vi "Stamp interface.vi"(4 "intercept":dbl=46.7 format="%.2f", 6 "slope":dbl=1.91 format="%.2f", 10 "Controls":T1 {"Pump speed" format="%.2f"}, 11 "Serial Port":refnum<visa-resource-name>) -> (0 "error out":errorcluster, 1 "too many items on":bool, 2 "Controls out":T1 {"Pump speed" format="%.2f"}, 3 "Serial Port out":refnum<visa-resource-name>)   [LabVIEW 2012]
uses:
  Stamp Controls.ctl
  switches.ctl
panel:
  out "on items":i16
  # "rpm"
  # "rpm"
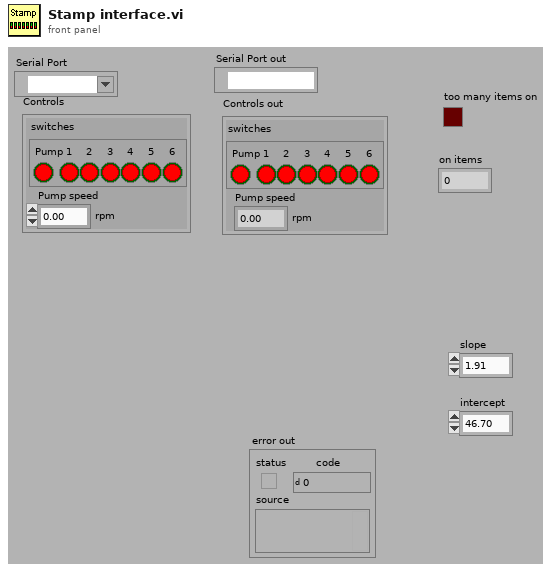
[diagram p1: front panel]
types:
  T1 = typedef "Stamp Controls.ctl" = cluster{"Pump speed":dbl, "switches":T2}
  T2 = typedef "switches.ctl" = cluster{"Pump":bool, "1":bool, "2":bool, "3":bool, "4":bool, "5":bool, "6":bool}
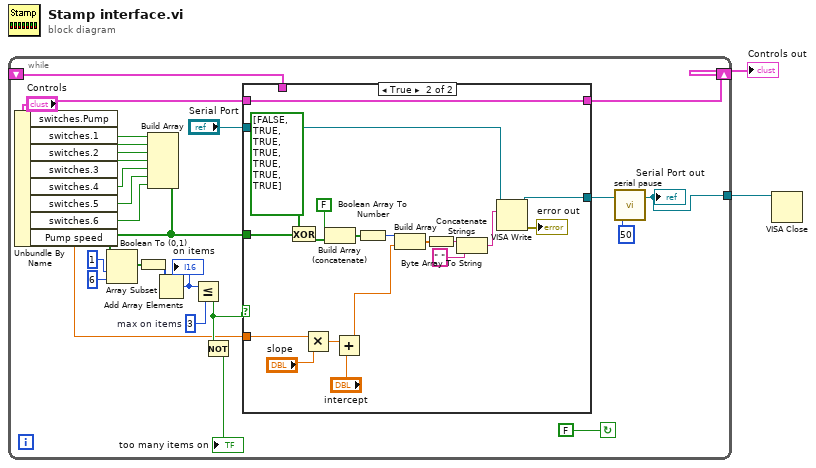
[diagram p0: block diagram]
diagram:
  n1 = while {
    shift-left: _ -> [w15]
    shift-right: [w16] -> w2
    tunnel: [w3] -> w1
    stop <- FALSE continue-if-true
    w23 = i16 3  # max on items
    n2 = Unbundle By Name("Controls") -> ("switches.Pump"=w7:bool, "switches.1"=w14:bool, "switches.2"=w13:bool, "switches.3"=w12:bool, "switches.4"=w11:bool, "switches.5"=w10:bool, "switches.6"=w9:bool, "Pump speed"=w19:dbl)
    n3 = Build Array(w7, w14, w13, w12, w11, w10, w9) -> (w8:bool[])
    n4 = Array Subset(array=w8, index=1 ("Array Index"), length=6 ("Array Length")) -> (w25:bool[])
    n5 = Boolean To (0,1)(Boolean=w25) -> (0, 1=w24:i16[])
    n6 = Add Array Elements(numeric array=w24) -> (sum=w22:i16)
    "on items" <- w22
    n7 = Less Or Equal?(x=w22, y=w23) -> (x <= y?=w20:bool)
    n8 = Not(x=w20) -> (.not. x?=→"too many items on":bool)
    n9 = case shown="True" w20 {
      tunnel: w8 -> [_ w38]
      tunnel: w19 -> [_ w35]
      tunnel: [w29 w34] -> w16
      tunnel: "Controls" -> [_ w34]
      tunnel: w15 -> [w29 _]
      tunnel: [w28 w31] -> w5
      tunnel: "Serial Port" -> [w28 w32]
      frame False {
      }
      frame True {
        n10 = Exclusive Or(1:w38, 2:bool[] [FALSE, TRUE, TRUE, TRUE, TRUE, TRUE, TRUE] ("inverting")) -> (0:w39:bool[])
        n11 = Multiply(x=w35, y="slope") -> (x*y=w44:dbl)
        n12 = Build Array (concatenate)(FALSE, w39) -> (w36:bool[])
        n13 = Add(x=w44, y="intercept") -> (x+y=w48:dbl)
        n14 = Boolean Array To Number(Boolean array=w36) -> (number=w45:u32)
        n15 = Build Array(w45, w48) -> (w41:dbl[])
        n16 = Byte Array To String(unsigned byte array=w41) -> (string=w46:string)
        n17 = Concatenate Strings(w46, " ") -> (w33:string)
        n18 = VISA Write(VISA resource name=w32, write buffer=w33) -> (VISA resource name out=w31:refnum<visa-resource-name>, error out=→"error out":errorcluster)  [unwired: 1 in, 1 out]
      }
    }
    n19 = call "serial pause.vi"("delay (ms)"=u32 50 ("millisecond multiple"), "Serial Port in"=w5) -> ("Serial Port out"=w3:refnum<visa-resource-name>)  [unwired: 1 in]
    "Serial Port out" <- w3
  }
  "Controls out" <- w2
  n20 = VISA Close(VISA resource name=w1) -> ()  [unwired: 1 in, 1 out]
